vi "Read remote_port .vi"(8 "error in (no error)":errorcluster, 11 "Socket.TCP in":refnum<class "Socket.TCP.lvclass">) -> (0 "error out":errorcluster, 2 "remote_port":u16, 3 "Socket.TCP out":refnum<class "Socket.TCP.lvclass">)   [LabVIEW 2014, in "Socket.lvlib" / "Socket.TCP.lvclass"]
uses:
  Socket.TCP.lvclass
  Socket.TCP.lvclass/Socket.TCP.ctl
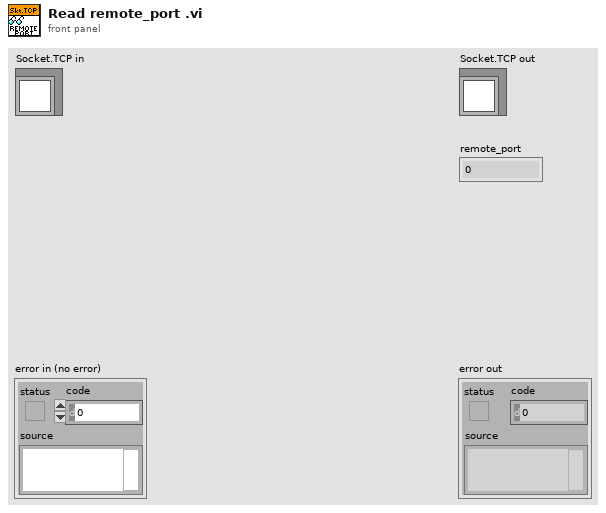
[diagram p1: front panel]
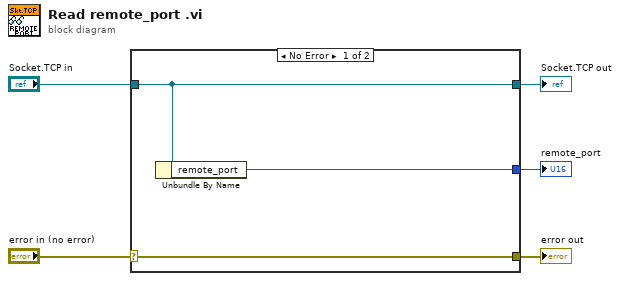
[diagram p0: block diagram]
diagram:
  n1 = case shown="No Error" "error in (no error)" {
    selector: "error in (no error)" -> [w8 w9]
    tunnel: [w8 w9] -> w4
    tunnel: [w7 w10] -> w2
    tunnel: "Socket.TCP in" -> [w7 w10]
    tunnel: [w6 _] -> w1
    frame No Error {
      n2 = Unbundle By Name(w7) -> ("remote_port"=w6:u16)
    }
    frame Error {
    }
  }
  "error out" <- w4
  "Socket.TCP out" <- w2
  "remote_port" <- w1
